vi "sv_Check for Weighting Conflict (spectrum).vi"(4 "existing weighting":T1 items=["Linear", "A-weighting", "B-weighting", "C-weighting", "ITU-R 468-4", "Dolby", "CCITT", "C-message", "Wb", "Wc", "Wd", "We", "Wf", "Wh", "Wj", "Wk", "Wm", "AES17 20 kHz lowpass", "AES17 40 kHz lowpass", "AES17 20 kHz highpass", "AES17 40 kHz highpass"], 6 "desired weighting":T1 items=["Linear", "A-weighting", "B-weighting", "C-weighting", "ITU-R 468-4", "Dolby", "CCITT", "C-message", "Wb", "Wc", "Wd", "We", "Wf", "Wh", "Wj", "Wk", "Wm", "AES17 20 kHz lowpass", "AES17 40 kHz lowpass", "AES17 20 kHz highpass", "AES17 40 kHz highpass"], 8 "error in (no error)":errorcluster) -> (0 "error out":errorcluster)   [LabVIEW 2017]
doc: "Make sure we will not be applying weighting twice if an external weighting filter has been used"
uses:
  <vilib>/addons/_NISVFA/_Shared subVIs/Controls/svc_Weighting Filter Text Ring.ctl
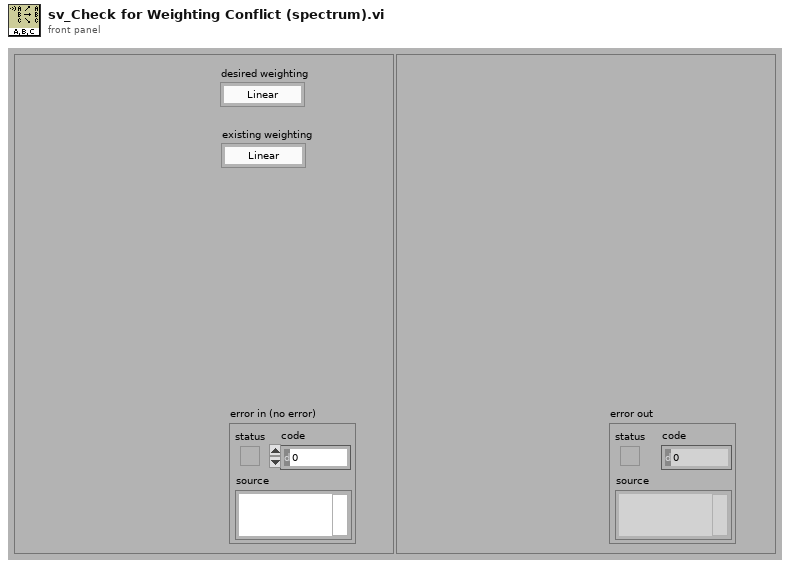
[diagram p1: front panel]
types:
  T1 = typedef "svc_Weighting Filter Text Ring.ctl" = u16
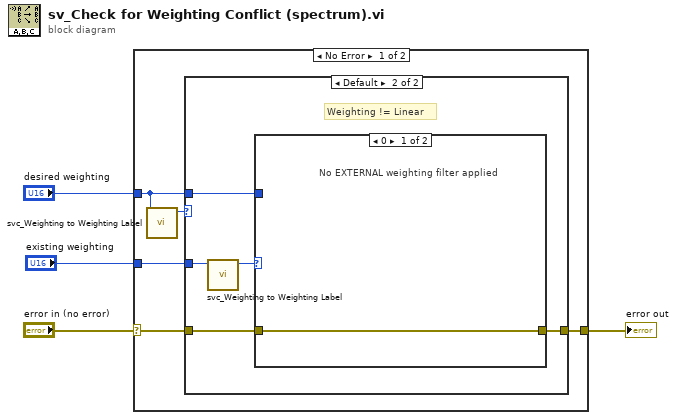
[diagram p0: block diagram]
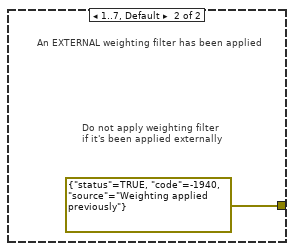
[diagram p3: hidden frame]
diagram:
  n1 = case shown="No Error" "error in (no error)" {
    selector: "error in (no error)" -> [w9 w18]
    tunnel: "desired weighting" -> [w6 _]
    tunnel: [w8 w18] -> w3
    tunnel: "existing weighting" -> [w5 _]
    frame No Error {
      n2 = call <vilib>:"svc_Weighting to Weighting Label.vi"("weighting filter"=w6) -> ("weighting enum"=w7:T1)  [unwired: 9 in, 1 out]
      n3 = case shown="Default" w7 {
        tunnel: w9 -> [w10 w11]
        tunnel: [w10 w15] -> w8
        tunnel: w6 -> [_ w14]
        tunnel: w5 -> [_ w12]
        frame 0 {
          # "Weighting = Linear...\ndo nothing"
        }
        frame Default {
          # "Weighting != Linear"
          n4 = call <vilib>:"svc_Weighting to Weighting Label.vi"("weighting filter"=w12) -> ("weighting enum"=w13:T1)  [unwired: 9 in, 1 out]
          n5 = case shown="0" w13 {
            tunnel: [w16 errorcluster {"status"=TRUE, "code"=-1940, "source"="Weighting applied previously"} ("error out")] -> w15
            tunnel: w14 -> [_ _]
            tunnel: w11 -> [w16 _]
            frame 0 {
              # "No EXTERNAL weighting filter applied"
            }
            frame 1..7, Default {
              # "Do not apply weighting filter\nif it's been applied externally"
              # "An EXTERNAL weighting filter has been applied"
            }
          }
        }
      }
    }
    frame Error {
    }
  }
  "error out" <- w3
